vi "Readout_Spectrum.vi"(0 "tdms file in":refnum<k34>, 1 "Fraction In":cluster{"X_in":dbl[], "Y_in":dbl[]}, 5 "Ch_in":T1, 9 "Spectrum?":bool, 11 "Intensity_in":i32[][](array[numeric]), 12 "group name":string, 13 "channel names":string[](array[string])) -> (3 "Fraction_out":T2, 4 "tdms file out":refnum<k34>, 6 "Ch_out":cluster{dbl[], dbl[], dbl[], dbl[]}, 14 "Spectrum_out":T3(array[cluster]), 15 "Intensity_out":i32[][](array[numeric]))   [LabVIEW 2019]
uses:
  SiPM_Tests_Global_Var.vi
  Agilent_lib/Public/Data/Read Measurement (Current Value).vi
  Agilent_lib/Agilent 2000 3000 X-Series.lvlib
  <vilib>/Analysis/NI_AALPro.lvlib
  <vilib>/gmath/NI_Gmath.lvlib
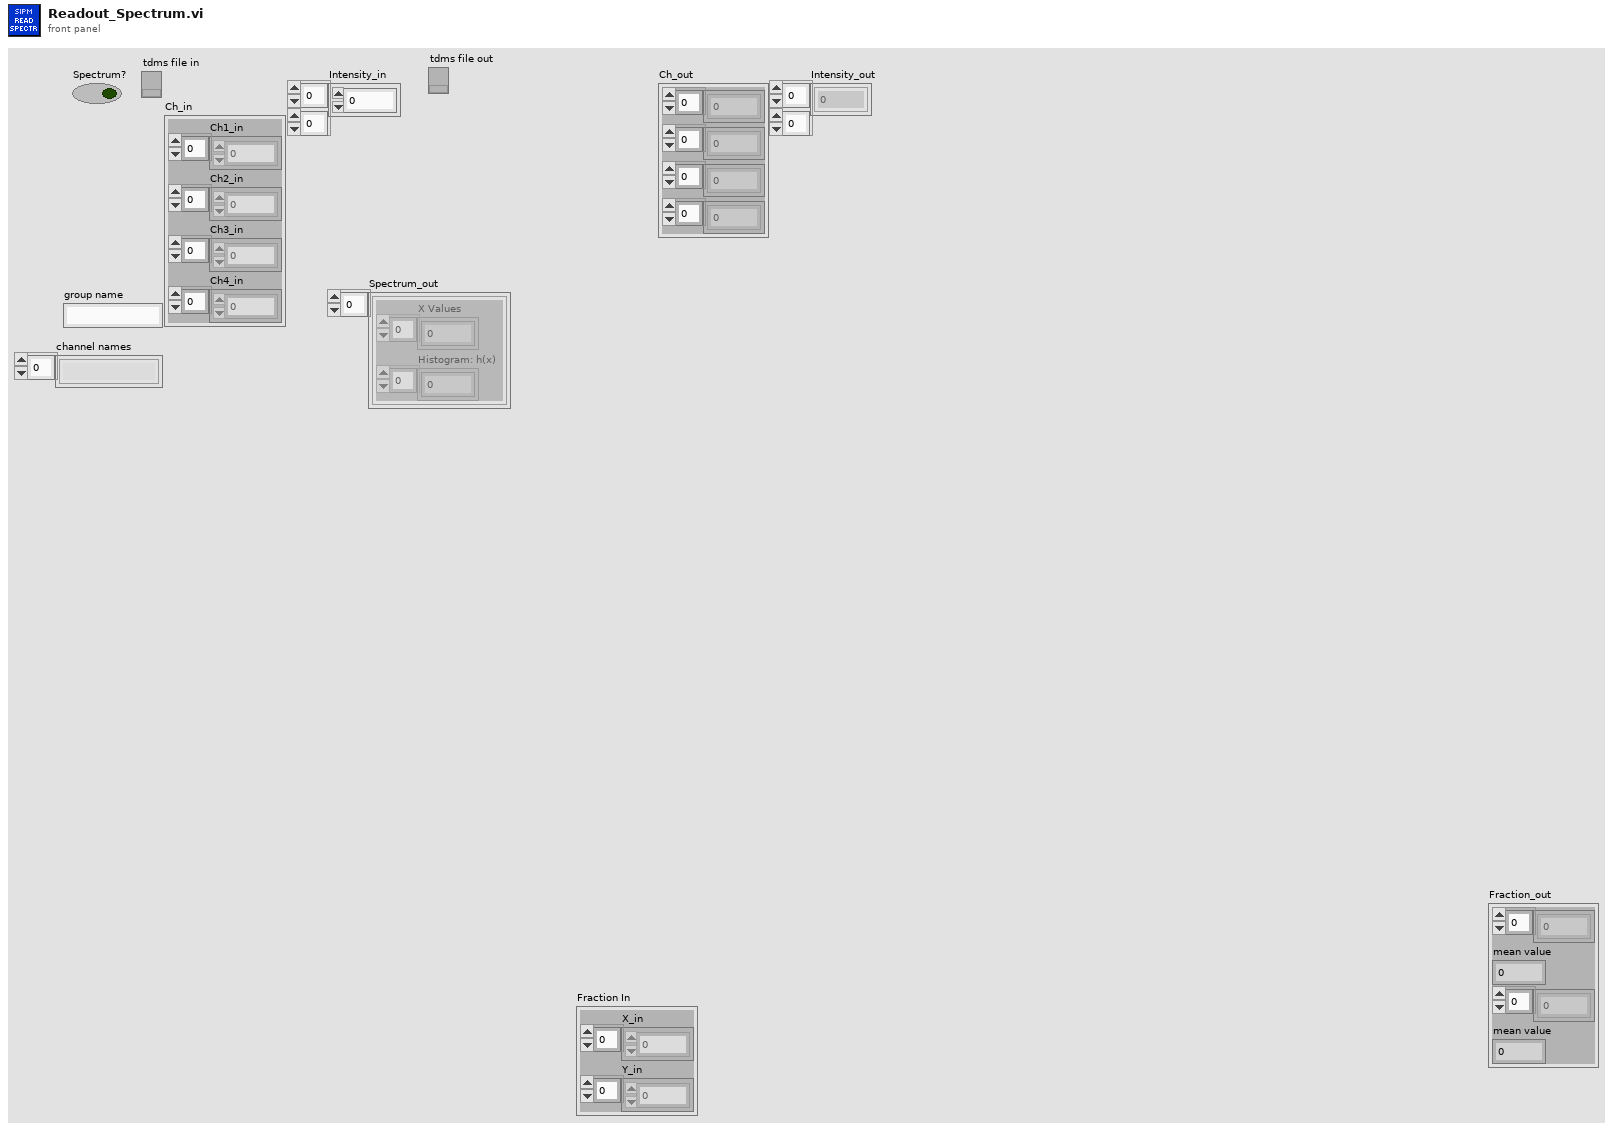
[diagram p1: front panel]
types:
  T1 = cluster{"Ch1_in":dbl[], "Ch2_in":dbl[], "Ch3_in":dbl[], "Ch4_in":dbl[]}
  T2 = cluster{dbl[], "mean value":dbl, dbl[], "mean value":dbl}
  T3 = cluster{"X Values":dbl[], "Histogram: h(x)":i32[]}[]
  T4 = cluster{"X Values":dbl[], "Histogram: h(x)":i32[]}
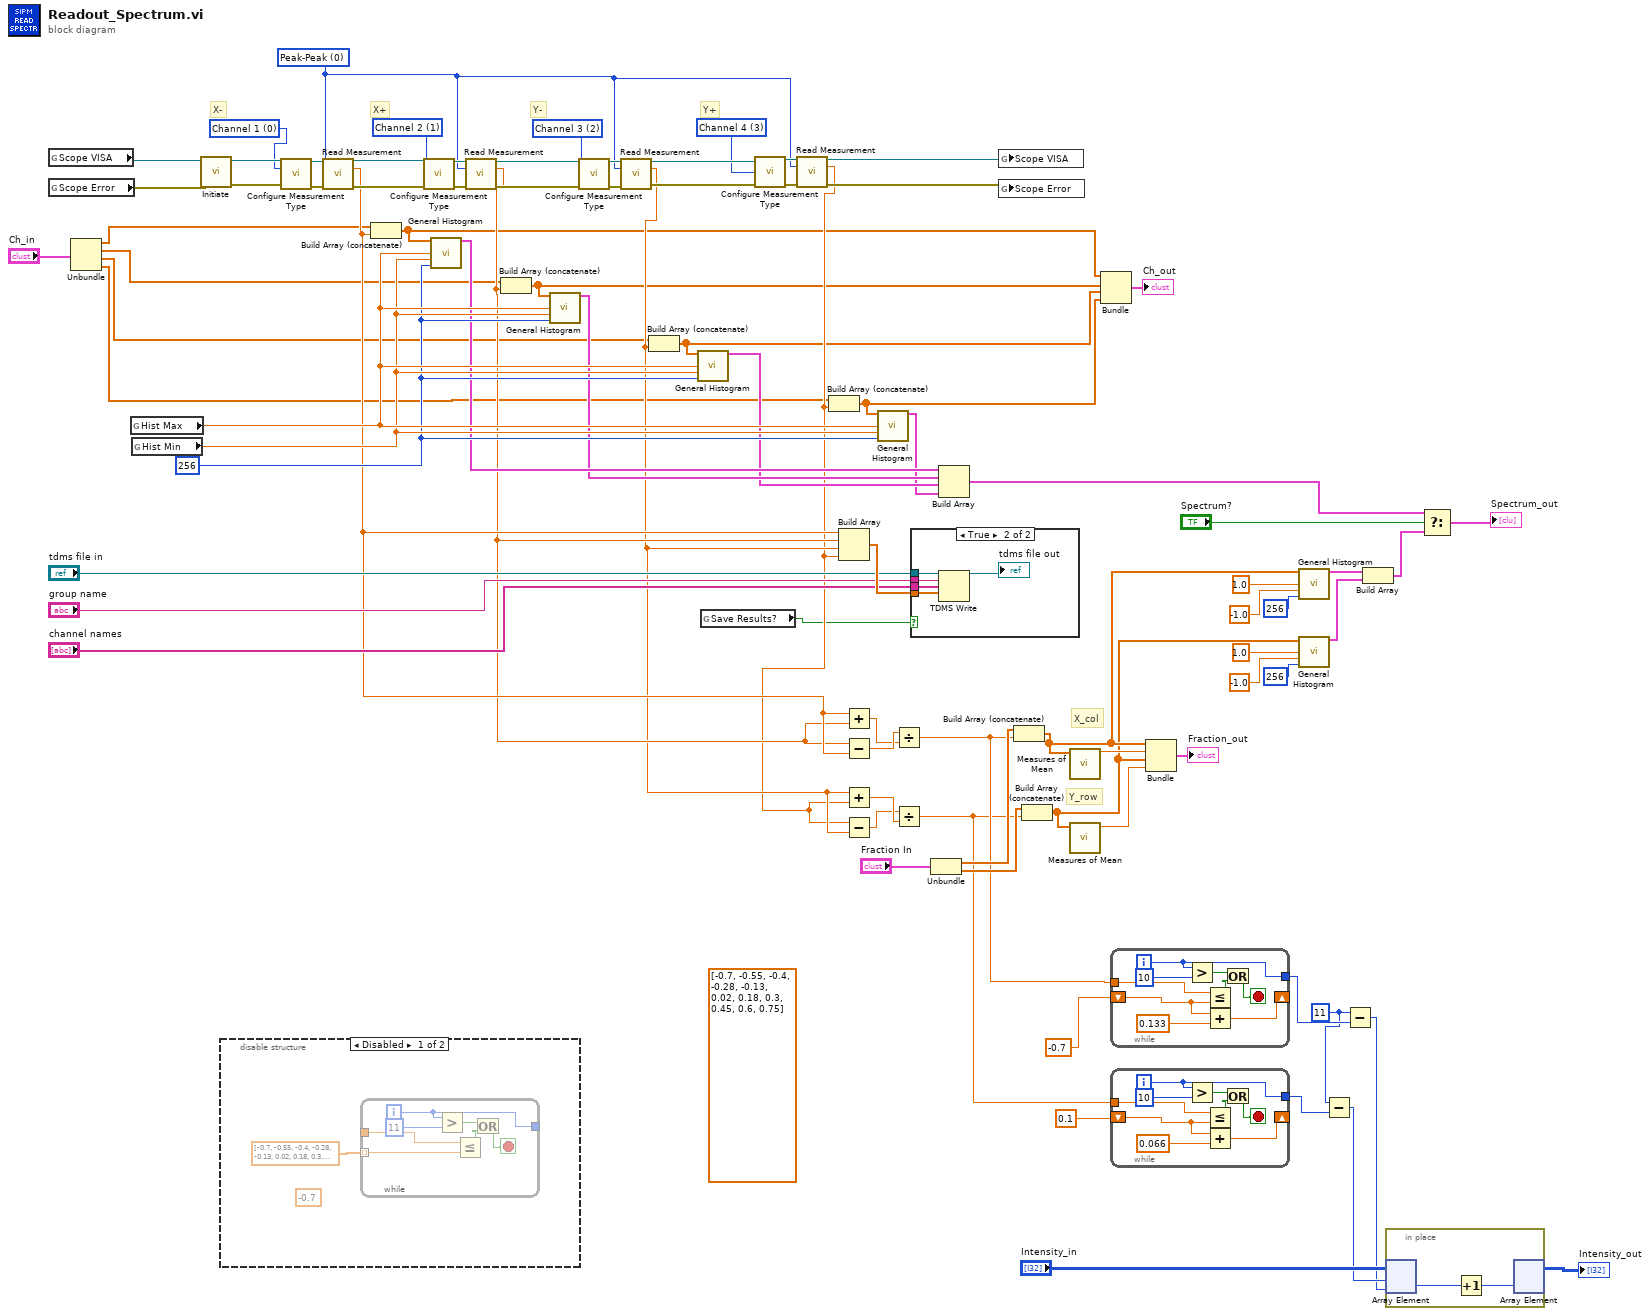
[diagram p0: block diagram]
diagram:
  w1 = 0 items=["Peak-Peak", "Maximum", "Mimimum", "Amplitude", "Top", "Base", "Overshoot", "Preshoot", "Average - N Cycles", "Average - Full Screen", "DC RMS - N Cycles", "DC RMS - Full Screen", "AC RMS - N Cycles", "AC RMS - Full Screen (Std Dev)", "Ratio", "Period", "Frequency", "Counter", "+Width", "-Width", "Burst Width", "Duty Cycle", "Rise Time", "Fall Time", "Delay", "Phase", "X minY", "X maxY", "Positive Pulse Count", "Negative Pulse Count", "Raising Edge Count", "Falling Edge Count", "Area - N Cycle", "Area - Full Screen", "Nth Edge Time", "Nth Edge Cross Level Time"] ("Measurement Type (0: Peak-Peak)")
  w4 = 11 ("x")
  (unwired) dbl[] [-0.7, -0.55, -0.4, -0.28, -0.13, 0.02, 0.18, 0.3, 0.45, 0.6, 0.75]
  w66 = 0 items=["Channel 1"=0, "Channel 2"=1, "Channel 3"=2, "Channel 4"=3, "Math"=4, "Waveform Memory 1"=5, "Waveform Memory 2"=6, "D0"=13, "D1"=14, "D2"=15, "D3"=16, "D4"=17, "D5"=18, "D6"=19, "D7"=20, "D8"=21, "D9"=22, "D10"=23, "D11"=24, "D12"=25, "D13"=26, "D14"=27, "D15"=28, "External"=29, "Function"=32] ("Measurement Source 1 (0: Channel 1)")
  w67 = 3 items=["Channel 1"=0, "Channel 2"=1, "Channel 3"=2, "Channel 4"=3, "Math"=4, "Waveform Memory 1"=5, "Waveform Memory 2"=6, "D0"=13, "D1"=14, "D2"=15, "D3"=16, "D4"=17, "D5"=18, "D6"=19, "D7"=20, "D8"=21, "D9"=22, "D10"=23, "D11"=24, "D12"=25, "D13"=26, "D14"=27, "D15"=28, "External"=29, "Function"=32] ("Measurement Source 1 (0: Channel 1)")
  w63 = 256 ("# bins")
  w82 = 2 items=["Channel 1"=0, "Channel 2"=1, "Channel 3"=2, "Channel 4"=3, "Math"=4, "Waveform Memory 1"=5, "Waveform Memory 2"=6, "D0"=13, "D1"=14, "D2"=15, "D3"=16, "D4"=17, "D5"=18, "D6"=19, "D7"=20, "D8"=21, "D9"=22, "D10"=23, "D11"=24, "D12"=25, "D13"=26, "D14"=27, "D15"=28, "External"=29, "Function"=32] ("Measurement Source 1 (0: Channel 1)")
  w77 = 1 items=["Channel 1"=0, "Channel 2"=1, "Channel 3"=2, "Channel 4"=3, "Math"=4, "Waveform Memory 1"=5, "Waveform Memory 2"=6, "D0"=13, "D1"=14, "D2"=15, "D3"=16, "D4"=17, "D5"=18, "D6"=19, "D7"=20, "D8"=21, "D9"=22, "D10"=23, "D11"=24, "D12"=25, "D13"=26, "D14"=27, "D15"=28, "External"=29, "Function"=32] ("Measurement Source 1 (0: Channel 1)")
  # "Y-"
  # "Y+"
  # "X-"
  # "X+"
  # "Y_row"
  # "X_col"
  n1 = global read "SiPM_Tests_Global_Var.vi" "Scope VISA"() -> (w83:refnum<visa-resource-name>)
  n2 = global read "SiPM_Tests_Global_Var.vi" "Scope Error"() -> (w84:errorcluster)
  n3 = Unbundle("Ch_in") -> ("Ch1_in"=w36:dbl[], "Ch2_in"=w35:dbl[], "Ch3_in"=w34:dbl[], "Ch4_in"=w33:dbl[])
  n4 = global read "SiPM_Tests_Global_Var.vi" "Hist Max"() -> (w65:dbl)
  n5 = global read "SiPM_Tests_Global_Var.vi" "Hist Min"() -> (w64:dbl)
  n6 = call "Initiate.vi"("error in (no error)"=w84, "VISA resource name"=w83) -> ("error out"=w85:errorcluster, "VISA resource name out"=w86:refnum<visa-resource-name>)  [unwired: 8 in]
  n7 = disable-structure shown="Disabled" {
    frame Disabled {
      (unwired) -0.7 ("y")
      n8 = while {
        tunnel: [w96] -> w87
        tunnel: [w92] -> w89
        tunnel: dbl[] [-0.7, -0.55, -0.4, -0.28, -0.13, 0.02, 0.18, 0.3, 0.45, 0.6, 0.75] -> [w90] mode=indexing
        i -> [w92]
        stop <- w95 stop-if-true
        n9 = Greater?(x=w92, y=11) -> (0:w93:bool)
        n10 = Less Or Equal?(x=w96, y=w90) -> (x <= y?=w94:bool)
        n11 = Or(x=w93, y=w94) -> (x .or. y?=w95:bool)
      }
    }
    frame Enabled {
    }
  }
  n12 = call "Configure Measurement Type.vi"("VISA resource name"=w86, "Measurement Type (0: Peak-Peak)"=w66, "error in (no error)"=w85) -> ("VISA resource name out"=w71:refnum<visa-resource-name>, "error out"=w72:errorcluster)  [unwired: 11 in]
  n13 = call-poly "Read Measurement.vi"("VISA resource name"=w71, "Measurement Type (0: Peak-Peak)"=w1, "error in (no error)"=w72) -> ("VISA resource name out"=w74:refnum<visa-resource-name>, "Result Value"=w42:dbl, "error out"=w75:errorcluster)  [unwired: 10 in]
  n14 = Build Array (concatenate)(w36, w42) -> (w32:dbl[])
  n15 = call "Configure Measurement Type.vi"("VISA resource name"=w74, "Measurement Source 1 (0: Channel 1)"=w77, "error in (no error)"=w75) -> ("VISA resource name out"=w76:refnum<visa-resource-name>, "error out"=w73:errorcluster)  [unwired: 11 in]
  n16 = call <vilib>:"General Histogram.vi"("X"=w32, "max"=w65, "min"=w64, "# bins"=w63) -> ("Histogram Graph"=w62:T4)  [unwired: 7 in, 4 out]
  n17 = call-poly "Read Measurement.vi"("VISA resource name"=w76, "Measurement Type (0: Peak-Peak)"=w1, "error in (no error)"=w73) -> ("VISA resource name out"=w78:refnum<visa-resource-name>, "Result Value"=w41:dbl, "error out"=w79:errorcluster)  [unwired: 10 in]
  n18 = Build Array (concatenate)(w35, w41) -> (w31:dbl[])
  n19 = call <vilib>:"General Histogram.vi"("X"=w31, "max"=w65, "min"=w64, "# bins"=w63) -> ("Histogram Graph"=w61:T4)  [unwired: 7 in, 4 out]
  n20 = call "Configure Measurement Type.vi"("VISA resource name"=w78, "Measurement Source 1 (0: Channel 1)"=w82, "error in (no error)"=w79) -> ("VISA resource name out"=w80:refnum<visa-resource-name>, "error out"=w81:errorcluster)  [unwired: 11 in]
  n21 = call-poly "Read Measurement.vi"("VISA resource name"=w80, "Measurement Type (0: Peak-Peak)"=w1, "error in (no error)"=w81) -> ("VISA resource name out"=w69:refnum<visa-resource-name>, "Result Value"=w40:dbl, "error out"=w68:errorcluster)  [unwired: 10 in]
  n22 = Build Array (concatenate)(w34, w40) -> (w30:dbl[])
  n23 = call <vilib>:"General Histogram.vi"("X"=w30, "max"=w65, "min"=w64, "# bins"=w63) -> ("Histogram Graph"=w60:T4)  [unwired: 7 in, 4 out]
  n24 = global read "SiPM_Tests_Global_Var.vi" "Save Results?"() -> (w38:bool)
  n25 = call "Configure Measurement Type.vi"("VISA resource name"=w69, "Measurement Source 1 (0: Channel 1)"=w67, "error in (no error)"=w68) -> ("VISA resource name out"=w70:refnum<visa-resource-name>, "error out"=w27:errorcluster)  [unwired: 11 in]
  n26 = call-poly "Read Measurement.vi"("VISA resource name"=w70, "Measurement Type (0: Peak-Peak)"=w1, "error in (no error)"=w27) -> ("VISA resource name out"=w58:refnum<visa-resource-name>, "Result Value"=w39:dbl, "error out"=w57:errorcluster)  [unwired: 10 in]
  n27 = Build Array (concatenate)(w33, w39) -> (w29:dbl[])
  n28 = Build Array(w42, w41, w40, w39) -> (w56:dbl[])
  n29 = Add(x=w42, y=w41) -> (x+y=w51:dbl)
  n30 = Subtract(x=w41, y=w42) -> (x-y=w52:dbl)
  n31 = Add(x=w40, y=w39) -> (x+y=w50:dbl)
  n32 = Subtract(x=w39, y=w40) -> (x-y=w49:dbl)
  n33 = call <vilib>:"General Histogram.vi"("X"=w29, "max"=w65, "min"=w64, "# bins"=w63) -> ("Histogram Graph"=w59:T4)  [unwired: 7 in, 4 out]
  n34 = Divide(x=w52, y=w51) -> (x/y=w9:dbl)
  n35 = Divide(x=w49, y=w50) -> (x/y=w6:dbl)
  n36 = case shown="True" w38 {
    tunnel: w56 -> [_ w101]
    tunnel: "tdms file in" -> [_ w99]
    tunnel: "group name" -> [_ w98]
    tunnel: "channel names" -> [_ w97]
    frame False {
    }
    frame True {
      n37 = TDMS Write(0:w99, 5:w98, 7:w97, 9:w101) -> (4:→"tdms file out":refnum<k34>)  [unwired: 2 in, 3 out]
    }
  }
  n38 = Unbundle("Fraction In") -> ("X_in"=w44:dbl[], "Y_in"=w43:dbl[])
  n39 = Build Array(w62, w61, w60, w59) -> (w17:T3)
  n40 = global write "SiPM_Tests_Global_Var.vi" "Scope VISA"(w58) -> ()
  n41 = global write "SiPM_Tests_Global_Var.vi" "Scope Error"(w57) -> ()
  n42 = Build Array (concatenate)(w44, w9) -> (w23:dbl[])
  n43 = Build Array (concatenate)(w43, w6) -> (w11:dbl[])
  n44 = call <vilib>:"Measures of Mean.vi"("x array"=w23) -> ("mean value"=w48:dbl)  [unwired: 9 in, 1 out]
  n45 = call <vilib>:"Measures of Mean.vi"("x array"=w11) -> ("mean value"=w47:dbl)  [unwired: 9 in, 1 out]
  n46 = Bundle(w32, w31, w30, w29) -> (→"Ch_out":cluster{dbl[], dbl[], dbl[], dbl[]})  [unwired: 1 in]
  n47 = while {
    tunnel: w9 -> [w110]
    shift-right: [w108] -> _
    shift-left: -0.7 ("y") -> [w109]
    tunnel: [w103] -> w7
    i -> [w103]
    stop <- w106 stop-if-true
    n48 = Greater?(x=w103, y=10) -> (0:w104:bool)
    n49 = Less Or Equal?(x=w110, y=w109) -> (x <= y?=w105:bool)
    n50 = Add(x=w109, y=0.133) -> (x+y=w108:dbl)
    n51 = Or(x=w104, y=w105) -> (x .or. y?=w106:bool)
  }
  n52 = while {
    tunnel: w6 -> [w119]
    shift-right: [w117] -> _
    shift-left: 0.1 ("y") -> [w118]
    tunnel: [w112] -> w5
    i -> [w112]
    stop <- w115 stop-if-true
    n53 = Greater?(x=w112, y=10) -> (0:w113:bool)
    n54 = Less Or Equal?(x=w119, y=w118) -> (x <= y?=w114:bool)
    n55 = Add(x=w118, y=0.066) -> (x+y=w117:dbl)
    n56 = Or(x=w113, y=w114) -> (x .or. y?=w115:bool)
  }
  n57 = Bundle(w23, "mean value"=w48, w11, "mean value"=w47) -> (→"Fraction_out":T2)  [unwired: 1 in]
  n58 = call <vilib>:"General Histogram.vi"("X"=w23, "max"=1.0, "min"=-1.0, "# bins"=256) -> ("Histogram Graph"=w19:T4)  [unwired: 7 in, 4 out]
  n59 = call <vilib>:"General Histogram.vi"("X"=w11, "max"=1.0, "min"=-1.0, "# bins"=256) -> ("Histogram Graph"=w10:T4)  [unwired: 7 in, 4 out]
  n60 = Subtract(x=w4, y=w5) -> (x-y=w3:i32)
  n61 = Subtract(x=w4, y=w7) -> (x-y=w2:i32)
  n62 = Build Array(w19, w10) -> (w18:T3)
  n63 = in-place {
    n64 = in-place-array #1("Intensity_in", w3, w2) -> (w121:i32)
    n65 = Increment(x=w121) -> (x+1=w120:i32)
    n66 = in-place-array #1(w120) -> (→"Intensity_out":i32[][])  [unwired: 2 out]
  }
  n67 = Select(t=w17, s="Spectrum?", f=w18) -> (s? t:f=→"Spectrum_out":T3)
